vi "Add Widget to Container.vi"(5 "Container":refnum<class "QWidget.lvclass">, 8 "Error In":errorcluster, 9 "Label":string, 10 "Widget":refnum<class "QWidget.lvclass">, 11 "Splitter Builder in":refnum<class "Splitter Builder.lvclass">) -> (0 "Error Out":errorcluster, 3 "Splitter Builder out":refnum<class "Splitter Builder.lvclass">)   [LabVIEW 2014, in "Dynamic GUI Composition and Management.lvlib" / "Splitter Builder.lvclass"]
doc: "Copyright (c) 2016 Sze Howe Koh\nThis code is licensed under the MIT license"
uses:
  Splitter Builder.lvclass
  src/LabVIEW/Qt Widgets/QWidget/QWidget.lvclass
  src/LabVIEW/Qt Widgets/QSplitter/QSplitter.lvclass
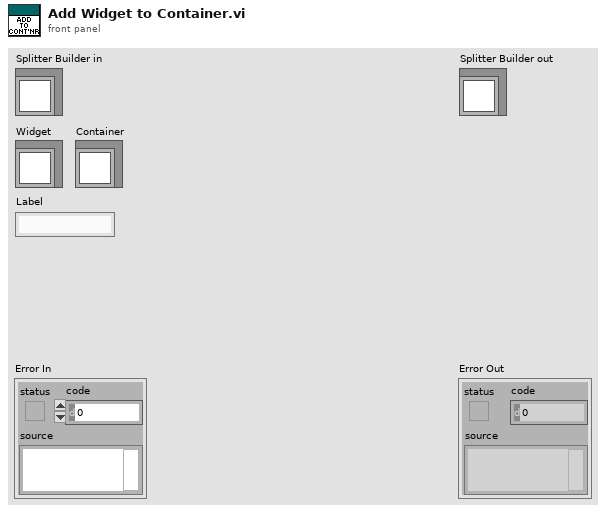
[diagram p1: front panel]
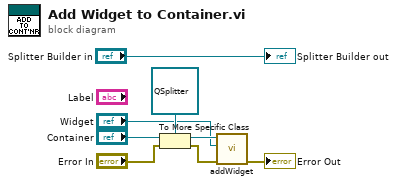
[diagram p0: block diagram]
diagram:
  n1 = To More Specific Class(target class=refnum<class "QSplitter.lvclass"> refnum ("QSplitter"), reference="Container", error in="Error In") -> (specific class reference=w3:refnum<class "QSplitter.lvclass">, error out=w4:errorcluster)
  n2 = call "addWidget.vi"("Error In"=w4, "widget"="Widget", "QSplitter In"=w3) -> ("Error Out"=→"Error Out":errorcluster)  [unwired: 7 in, 1 out]
  "Splitter Builder out" <- "Splitter Builder in"
